vi "데이터(4) 저장_상태벡터  txt파일로 저장.vi"(0 "Location":path, 1 "Data4":dbl, 2 "Data3":dbl, 3 "Data2":dbl, 4 "Data1":dbl) -> ()   [LabVIEW 2016]
panel:
  out "Combined Data":string
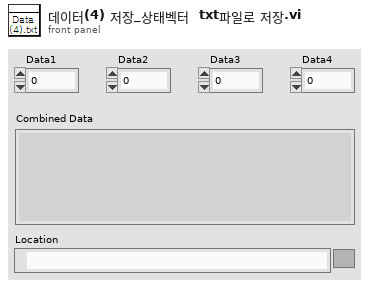
[diagram p1: front panel]
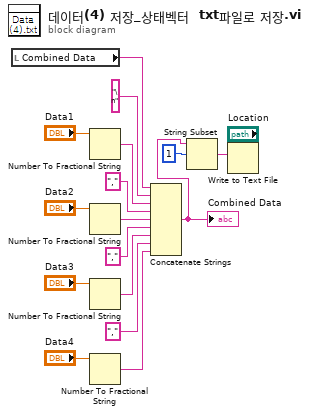
[diagram p0: block diagram]
diagram:
  n1 = local read "Combined Data"() -> (w4:string)
  n2 = Number To Fractional String(number="Data1") -> (F-format string=w16:string)  [unwired: 3 in]
  n3 = Number To Fractional String(number="Data2") -> (F-format string=w15:string)  [unwired: 3 in]
  n4 = Number To Fractional String(number="Data3") -> (F-format string=w8:string)  [unwired: 3 in]
  n5 = Number To Fractional String(number="Data4") -> (F-format string=w6:string)  [unwired: 3 in]
  n6 = Concatenate Strings ("문자열 연결")(w4, "\n" ("문자열"), w16, "," ("문자열"), w15, "," ("문자열"), w8, "," ("문자열"), w6) -> (w3:string)
  "Combined Data" <- w3
  n7 = String Subset(string=w3, offset (0)=1 ("오프셋(0)")) -> (substring=w2:string)  [unwired: 1 in]
  n8 = Write to Text File(file (use dialog)="Location", text=w2) -> ()  [unwired: 2 in, 3 out]
